vi "Autotest.vi"(8 "error in (no error)":errorcluster caption="entrée d'erreur (pas d'erreur)", 11 "Class Balance_Adam_GBK en entrée":refnum<class "Class Balance_Adam_GBK.lvclass">) -> (0 "error out":errorcluster caption="sortie d'erreur", 2 "Autotest Ok ?":bool, 3 "Class Balance_Adam_GBK en sortie":refnum<class "Class Balance_Adam_GBK.lvclass">)   [LabVIEW 2020, in "Library Instrument & Equipement.lvlib" / "Library Balance.lvlib" / "Class Balance_Adam_GBK.lvclass"]
uses:
  Class Balance_Adam_GBK.lvclass
  C:/Users/ngarcin/OneDrive - Altyor/Standard TB/Class/Balance/Balance (Default)/Class Balance (Default).lvclass
  <vilib>/Instr/_visa.llb/VISA Find Search Mode.ctl
  Balance (Default)/Class Balance (Default).lvclass
  Class Balance_Adam_GBK.lvclass/Class Balance_Adam_GBK.ctl
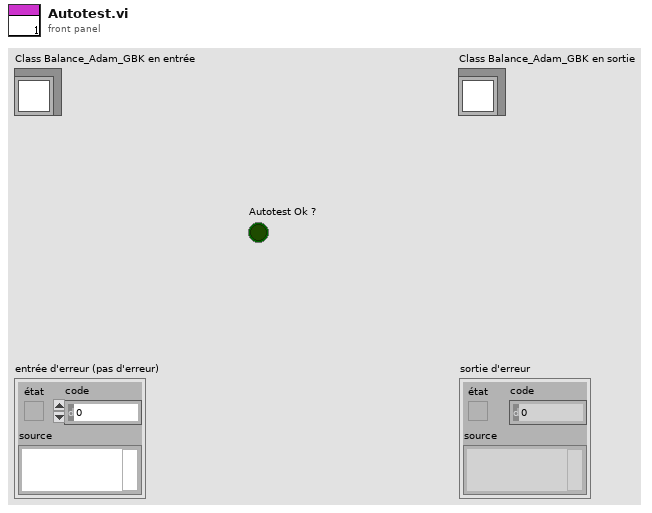
[diagram p1: front panel]
types:
  T1 = typedef "VISA Find Search Mode.ctl" = u32
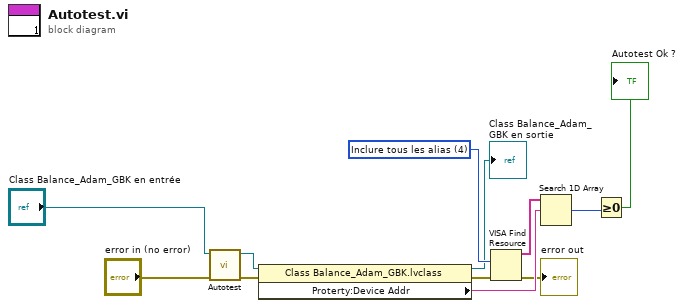
[diagram p0: block diagram]
diagram:
  w9 = T1 4 items=["Noms canoniques uniquement"=0, "Alias uniquement"=2, "Inclure les alias correspondants"=3, "Inclure tous les alias"=4] ("Search Mode")
  n1 = call-parent "Autotest.vi"("error in (no error)"="error in (no error)", "Class Balance (Default) en entrée"="Class Balance_Adam_GBK en entrée") -> ("error out"=w4:errorcluster, "Class Balance (Default) en sortie"=w5:refnum<class "Class Balance_Adam_GBK.lvclass">)  [unwired: 7 in, 1 out]
  n2 = property class="Class Balance_Adam_GBK.lvclass"(reference=w5, error in=w4) -> (reference out=→"Class Balance_Adam_GBK en sortie":refnum<class "Class Balance_Adam_GBK.lvclass">, error out=w10:errorcluster, "Proterty:Device Addr"=w8:string)
  n3 = VISA Find Resource(8:w10, 10:w9) -> (0:→"error out":errorcluster, 3:w7:string[])  [unwired: 1 in, 1 out]
  n4 = Search 1D Array(1D array=w7, element=w8) -> (index of element=w2:i32)  [unwired: 1 in]
  n5 = Greater Or Equal To 0?(x=w2) -> (x >= 0?=→"Autotest Ok ?":bool)
